vi "Smooth.vi"(8 "Error In":errorcluster caption="error in (no error)", 10 "Raw Signal Waveform In":waveform(dbl)) -> (0 "Error Out":errorcluster caption="error out", 2 "Smooth Signal Waveform Out":waveform(dbl))   [LabVIEW 2025]
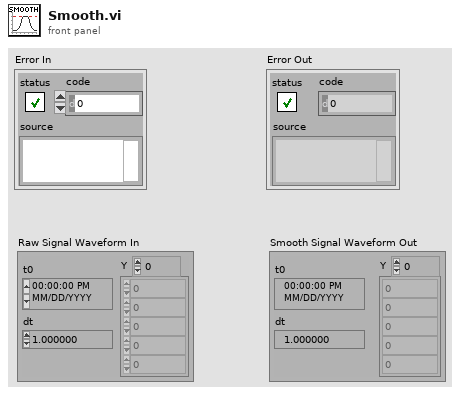
[diagram p1: front panel]
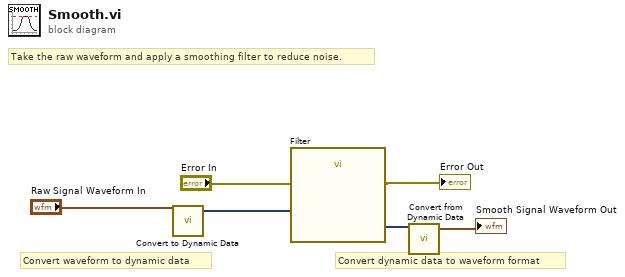
[diagram p0: block diagram]
diagram:
  # "Convert waveform to dynamic data"
  # "Convert dynamic data to waveform format"
  # "Take the raw waveform and apply a smoothing filter to reduce noise."
  n1 = call "Convert to Dynamic Data"("Waveform"="Raw Signal Waveform In") -> ("Dynamic Data Type"=w5:dynamicdata)  [unwired: 3 in]
  n2 = call "Filter"("error in (no error)"="Error In", "Signal"=w5) -> ("error out"=→"Error Out":errorcluster, "Filtered Signal"=w4:dynamicdata)  [unwired: 8 in]
  n3 = call "Convert from Dynamic Data"("Dynamic Data Type"=w4) -> ("Waveform"=→"Smooth Signal Waveform Out":waveform(dbl))  [unwired: 3 in]
